vi "方块数据.vi"() -> (3 "输出簇":T1)   [LabVIEW 2012]
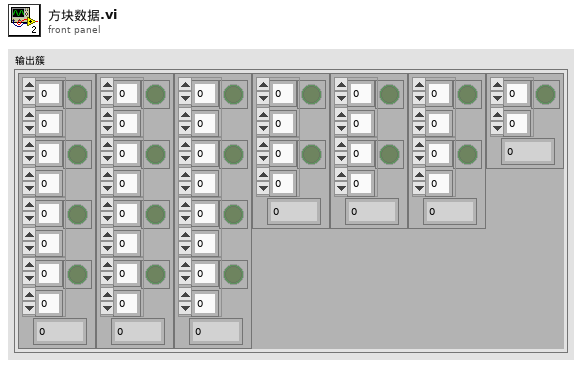
[diagram p1: front panel]
types:
  T1 = cluster{cluster{bool[][], bool[][], bool[][], bool[][], u32}, cluster{bool[][], bool[][], bool[][], bool[][], u32}, cluster{bool[][], bool[][], bool[][], bool[][], u32}, cluster{bool[][], bool[][], u32}, cluster{bool[][], bool[][], u32}, cluster{bool[][], bool[][], u32}, cluster{bool[][], u32}}
  T2 = cluster{bool[][], bool[][], bool[][], bool[][], u32}
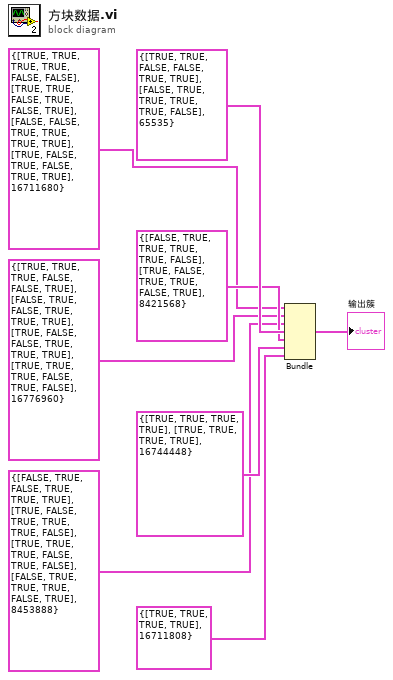
[diagram p0: block diagram]
diagram:
  n1 = Bundle(T2 {[[TRUE, TRUE, TRUE], [TRUE, FALSE, FALSE]], [[TRUE, TRUE], [FALSE, TRUE], [FALSE, TRUE]], [[FALSE, FALSE, TRUE], [TRUE, TRUE, TRUE]], [[TRUE, FALSE], [TRUE, FALSE], [TRUE, TRUE]], 16711680}, T2 {[[TRUE, TRUE, TRUE], [FALSE, FALSE, TRUE]], [[FALSE, TRUE], [FALSE, TRUE], [TRUE, TRUE]], [[TRUE, FALSE, FALSE], [TRUE, TRUE, TRUE]], [[TRUE, TRUE], [TRUE, FALSE], [TRUE, FALSE]], 16776960}, T2 {[[FALSE, TRUE, FALSE], [TRUE, TRUE, TRUE]], [[TRUE, FALSE], [TRUE, TRUE], [TRUE, FALSE]], [[TRUE, TRUE, TRUE], [FALSE, TRUE, FALSE]], [[FALSE, TRUE], [TRUE, TRUE], [FALSE, TRUE]], 8453888}, cluster{bool[][], bool[][], u32} {[[TRUE, TRUE, FALSE], [FALSE, TRUE, TRUE]], [[FALSE, TRUE], [TRUE, TRUE], [TRUE, FALSE]], 65535}, cluster{bool[][], bool[][], u32} {[[FALSE, TRUE, TRUE], [TRUE, TRUE, FALSE]], [[TRUE, FALSE], [TRUE, TRUE], [FALSE, TRUE]], 8421568}, cluster{bool[][], bool[][], u32} {[[TRUE, TRUE, TRUE, TRUE]], [[TRUE], [TRUE], [TRUE], [TRUE]], 16744448}, cluster{bool[][], u32} {[[TRUE, TRUE], [TRUE, TRUE]], 16711808}) -> (→"输出簇":T1)  [unwired: 1 in]
